vi "Stage_move_to_destination.vi"(8 "error IN":errorcluster, 10 "Stage position IN":T1={"X Position"=-23.0, "Y Position"=-18.0, "Z Position"=0.0}, 11 "reference IN":refnum<k7>) -> (0 "error OUT":errorcluster, 2 "Stage position OUT":T1={"X Position"=-23.0, "Y Position"=-18.0, "Z Position"=0.0}, 3 "reference OUT":refnum<k7>)   [LabVIEW 2020]
uses:
  typedefs/typedef_stage_position.ctl
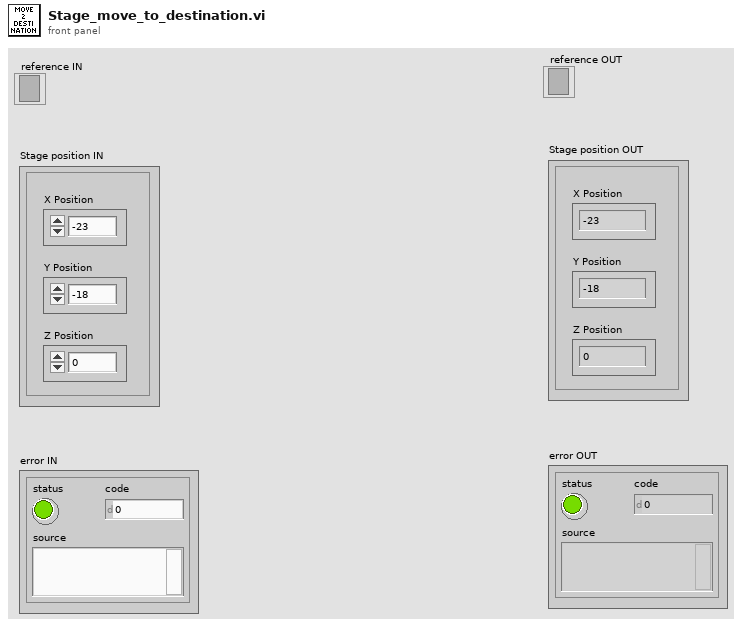
[diagram p1: front panel]
types:
  T1 = typedef "typedef_stage_position.ctl" = cluster{"X Position":dbl, "Y Position":dbl, "Z Position":dbl}
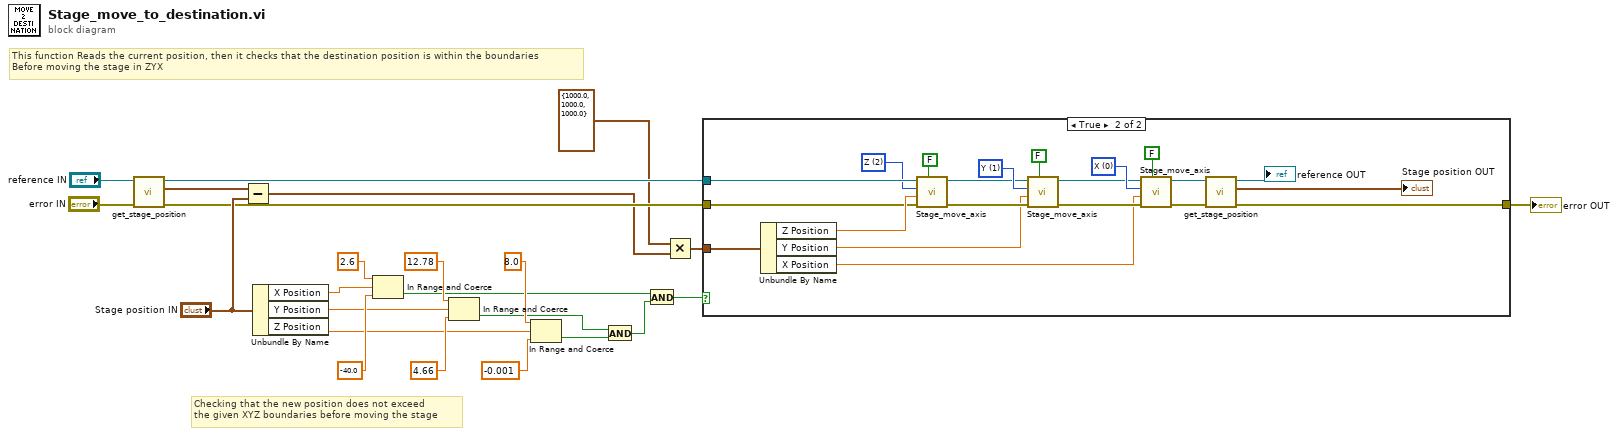
[diagram p0: block diagram]
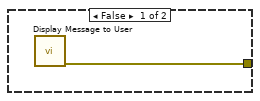
[diagram p2: hidden frame]
diagram:
  # "This function Reads the current position, then it checks that the destination position is within the boundaries\nBefore moving the stage in ZYX"
  # "Checking that the new position does not exceed \nthe given XYZ boundaries before moving the stage"
  n1 = call "get_stage_position.vi"("error IN"="error IN", "reference IN"="reference IN") -> ("error OUT"=w3:errorcluster, "Stage position OUT"=w23:T1, "reference OUT"=w24:refnum<k7>)  [unwired: 7 in]
  n2 = Subtract(x=w23, y="Stage position IN") -> (x-y=w1:T1)
  n3 = Unbundle By Name("Stage position IN") -> ("X Position"=w20:dbl, "Y Position"=w15:dbl, "Z Position"=w12:dbl)
  n4 = In Range and Coerce(upper limit=2.6, x=w20, lower limit=-40.0) -> (In Range?=w7:bool)  [unwired: 1 out]
  n5 = In Range and Coerce(upper limit=12.78, x=w15, lower limit=4.66) -> (In Range?=w9:bool)  [unwired: 1 out]
  n6 = In Range and Coerce(upper limit=8.0, x=w12, lower limit=-0.001) -> (In Range?=w10:bool)  [unwired: 1 out]
  n7 = And(x=w9, y=w10) -> (x .and. y?=w8:bool)
  n8 = And(x=w7, y=w8) -> (x .and. y?=w5:bool)
  n9 = Multiply(x=T1 {"X Position"=1000.0, "Y Position"=1000.0, "Z Position"=1000.0} ("y"), y=w1) -> (x*y=w11:T1)
  n10 = case shown="True" w5 {
    tunnel: w24 -> [_ w46]
    tunnel: w3 -> [_ w29]
    tunnel: w11 -> [_ w27]
    tunnel: [w25 w26] -> w6
    frame False {
      n11 = call "Display Message to User"() -> ("error out"=w25:errorcluster)  [unwired: 10 in, 1 out]
    }
    frame True {
      w39 = u16 0 items=["X", "Y", "Z"] ("Axes Select")
      w43 = u16 1 items=["X", "Y", "Z"] ("Axes Select")
      w45 = u16 2 items=["X", "Y", "Z"] ("Axes Select")
      n12 = Unbundle By Name(w27) -> ("Z Position"=w44:dbl, "Y Position"=w40:dbl, "X Position"=w34:dbl)
      n13 = call "Stage_move_axis.vi"("Direction true means positive increment"=FALSE, "error in (no error)"=w29, "Distance micrometer"=w44, "Axes Select"=w45, "reference IN"=w46) -> ("error OUT"=w41:errorcluster, "reference OUT"=w42:refnum<k7>)  [unwired: 5 in]
      n14 = call "Stage_move_axis.vi"("Direction true means positive increment"=FALSE, "error in (no error)"=w41, "Distance micrometer"=w40, "Axes Select"=w43, "reference IN"=w42) -> ("error OUT"=w38:errorcluster, "reference OUT"=w37:refnum<k7>)  [unwired: 5 in]
      n15 = call "Stage_move_axis.vi"("Direction true means positive increment"=FALSE, "error in (no error)"=w38, "Distance micrometer"=w34, "Axes Select"=w39, "reference IN"=w37) -> ("error OUT"=w35:errorcluster, "reference OUT"=w36:refnum<k7>)  [unwired: 5 in]
      n16 = call "get_stage_position.vi"("error IN"=w35, "reference IN"=w36) -> ("error OUT"=w26:errorcluster, "Stage position OUT"=→"Stage position OUT":T1, "reference OUT"=→"reference OUT":refnum<k7>)  [unwired: 7 in]
    }
  }
  "error OUT" <- w6
